vi "Engine-RPC-PWM-A-PID-Host.vi"() -> ()   [LabVIEW 2016]
uses:
  <vilib>/addons/Software Calibration Management/XControls/TBL1D.xctl
panel:
  in  "_ModeTab":enum32{"IMV PID", "HPV Lookup Table"}(tab)
  out "PWM-A_IMV_TdOut":sgl(slide) caption="IMV_ Td Action" max=0 scale=0.0..100.0 scale format="%#.2f"
  out "PWM-A_IMV_TiOut":sgl(slide) caption="IMV_ Ti Action" max=0 scale=0.0..100.0 scale format="%#.2f"
  out "PWM-A_IMV_KpOut":sgl(slide) caption="IMV_ Kc Action" max=0 scale=0.0..100.0 scale format="%#.2f"
  in  "PWM-A_IMV_PIDMin":sgl caption="[%]" format="%#.2f"
  in  "PWM-A_IMV_PIDMax":sgl caption="[%]" max=50 format="%#.2f"
  in  "PWM-A_IMV_Td":sgl caption="[]" format="%#.2f"
  in  "PWM-A_IMV_Ti":sgl caption="[]" format="%#.2f"
  in  "PWM-A_IMV_Kp":sgl caption="[%/bar]" format="%#.2f"
  in  "PWM-A_IMV_PIDFF":sgl caption="[]" format="%#.2f"
  out "PWM-A_IMVPID_Out":sgl caption="[%]" max=50
  in  "PWM-A_IMV_NonPIDFF":sgl caption="[]" format="%#.2f"
  in  "PWM-A_HPVDutyCyc_Tbl":cluster{"X":sgl[], "Y":sgl[]}(xcontrol) caption="[%]"
  # "+"
  # "OR"
  # "Pressure Setpoint\n[unit]"
  # "Duty Cycle\n[%]"
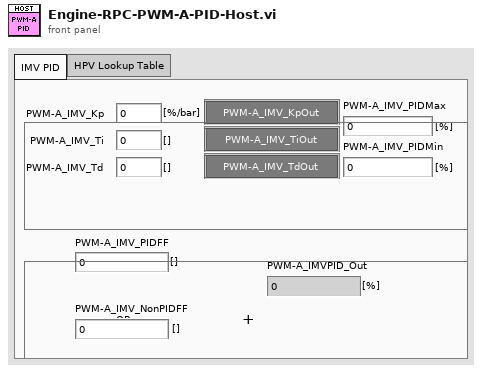
[diagram p1: front panel]
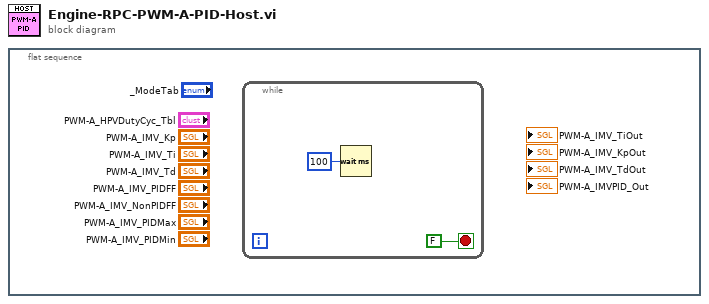
[diagram p0: block diagram]
diagram:
  n1 = flat-sequence {
    frame #0 {
      n2 = while {
        stop <- FALSE stop-if-true
        n3 = Wait (ms)(milliseconds to wait=u32 100) -> ()  [unwired: 1 out]
      }
    }
  }
